vi "MB ViRefCount.vi"(7 "Function":T1, 11 "reference ID":refnum<vi>) -> (2 "IDs":refnum<vi>[](array[refnum]), 3 "VI Running?":bool)   [LabVIEW 2019, in "NI_modbus_upd.lvlib"]
uses:
  Ctl/MB ViRefCount Function.ctl
  NI_modbus_upd.lvlib
panel:
  # "VI Name: MB RefCount.vi\nPurpose: Keep track of connection ID references."
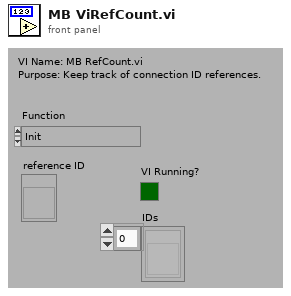
[diagram p1: front panel]
types:
  T1 = typedef "NI_modbus_upd.lvlib/MB ViRefCount Function.ctl" = enum16{"Init", "Add", "Remove", "Is Running?", "GetAll_IDs"}
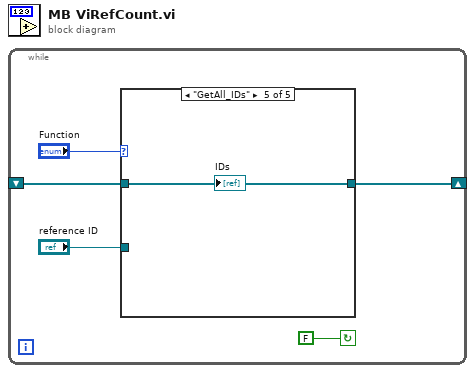
[diagram p0: block diagram]
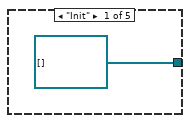
[diagram p2: hidden frame]
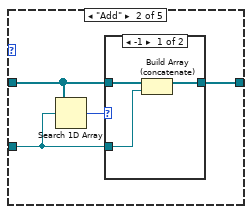
[diagram p3: hidden frame]
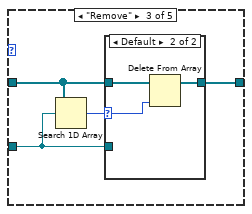
[diagram p5: hidden frame]
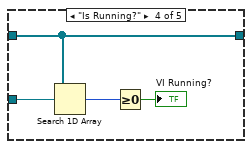
[diagram p7: hidden frame]
diagram:
  n1 = while {
    shift-right: [w4] -> _
    shift-left: _ -> [w3]
    stop <- FALSE continue-if-true
    n2 = case shown="\"GetAll_IDs\"" "Function" {
      tunnel: [refnum<vi>[] [] w8 w16 w25 w27] -> w4
      tunnel: w3 -> [_ w9 w17 w25 w27]
      tunnel: "reference ID" -> [_ w7 w15 w26 _]
      frame "Init" {
      }
      frame "Add" {
        n3 = Search 1D Array(1D array=w9, element=w7) -> (index of element=w10:i32)  [unwired: 1 in]
        n4 = case shown="-1" w10 {
          tunnel: [w11 w14] -> w8
          tunnel: w9 -> [w13 w14]
          tunnel: w7 -> [w12 _]
          frame -1 {
            n5 = Build Array (concatenate)(w13, w12) -> (w11:refnum<vi>[])
          }
          frame Default {
          }
        }
      }
      frame "Remove" {
        n6 = Search 1D Array(1D array=w17, element=w15) -> (index of element=w18:i32)  [unwired: 1 in]
        n7 = case shown="Default" w18 {
          selector: w18 -> [_ w21]
          tunnel: [w19 w20] -> w16
          tunnel: w17 -> [w19 w22]
          tunnel: w15 -> [_ _]
          frame -1 {
          }
          frame Default {
            n8 = Delete From Array(array=w22, index=w21) -> (array with subset deleted=w20:refnum<vi>[])  [unwired: 1 in, 1 out]
          }
        }
      }
      frame "Is Running?" {
        n9 = Search 1D Array(1D array=w25, element=w26) -> (index of element=w24:i32)  [unwired: 1 in]
        n10 = Greater Or Equal To 0?(x=w24) -> (x >= 0?=→"VI Running?":bool)
      }
      frame "GetAll_IDs" {
        "IDs" <- w27
      }
    }
  }
